vi "TDC_errorHandler.vi"(8 "Error In":errorcluster, 11 "TDC Return Code":i32) -> (0 "Error Out":errorcluster)   [LabVIEW 2011]
uses:
  tdcbase.dll
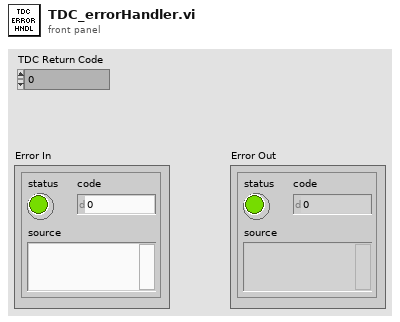
[diagram p1: front panel]
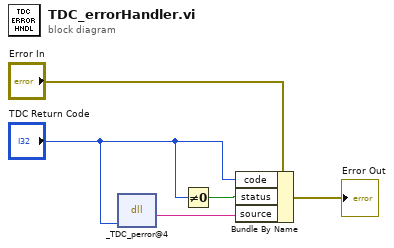
[diagram p0: block diagram]
diagram:
  n1 = dll-call lib="X:/tdcbase.dll" fn="_TDC_perror@4"("rc"="TDC Return Code") -> ("return type"=w1:string)  [unwired: 4 in, 2 out]
  n2 = Not Equal To 0?(x="TDC Return Code") -> (x != 0?=w5:bool)
  n3 = Bundle By Name(cluster="Error In", "code"="TDC Return Code", "status"=w5, "source"=w1) -> (→"Error Out":errorcluster)
